vi "Export To File.vi"(4 "Always Overwrite":bool, 6 "Hide Grid":bool, 7 "Control Ref Queue":T1, 8 "error in (no error)":errorcluster, 9 "Path":path, 10 "Target":enum32{"File", "Clipboard"}(ring), 11 "File Type":enum32{"BMP", "EPS", "EMF", "PICT"}(ring)) -> (0 "error out":errorcluster)   [LabVIEW 2017, in "XY Plot Matrix.lvclass"]
uses:
  <vilib>/Math Plots/2D Math Plots/XY Plot Matrix/XY Plot Matrix/XY Plot Matrix.lvclass
  <vilib>/Math Plots/2D Math Plots/2D Plot/Action String/XYPlotMatrix Ctrl Act Queue.ctl
  <vilib>/Math Plots/2D Math Plots/2D Plot/Action String/XYPlotMatrix Ctrl Act Cluster.ctl
  <vilib>/Math Plots/2D Math Plots/2D Plot/Action String/2DMathPlot State Class.ctl
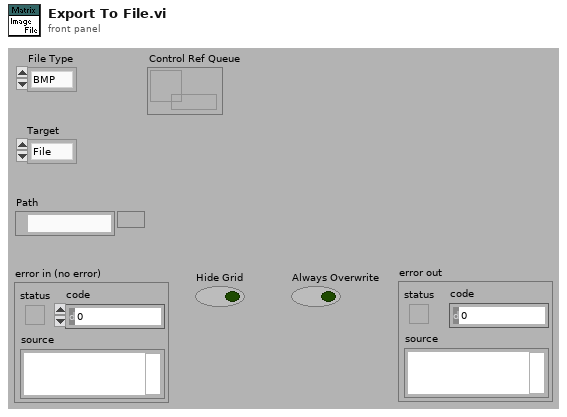
[diagram p1: front panel]
types:
  T1 = typedef "XYPlotMatrix Ctrl Act Queue.ctl" = refnum<queue>
  T2 = typedef "XYPlotMatrix Ctrl Act Cluster.ctl" = cluster{"Facade VI":refnum<vi>, "XControl":refnum<vi>, "Sub Panel":refnum<vi>, "Sub VI":refnum<vi>, "Export Image":refnum<vi>, "Display State Change Class":T3}
  T3 = typedef "2DMathPlot State Class.ctl" = enum16{"Update All (Undo)", "Update General", "Update Appearance", "Update Format", "Update Scale", "Update Marker", "Update Cursor", "None"}
  T4 = typedef "LVBoundsTypeDef.ctl" = cluster{"Width":u32, "Height":u32}
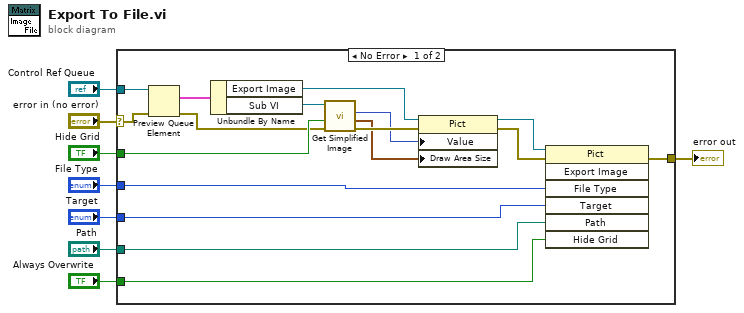
[diagram p0: block diagram]
diagram:
  n1 = case shown="No Error" "error in (no error)" {
    selector: "error in (no error)" -> [w11 w26]
    tunnel: "Hide Grid" -> [w21 _]
    tunnel: "Target" -> [w18 _]
    tunnel: "Path" -> [w17 _]
    tunnel: "File Type" -> [w9 _]
    tunnel: "Control Ref Queue" -> [w16 _]
    tunnel: [w13 w26] -> w3
    tunnel: "Always Overwrite" -> [w10 _]
    frame No Error {
      n2 = Preview Queue Element(queue=w16, error in (no error)=w11) -> (element=w15:T2, error out=w20:errorcluster)  [unwired: 3 out]
      n3 = Unbundle By Name(w15) -> ("Export Image"=w12:refnum<vi>, "Sub VI"=w19:refnum<vi>)
      n4 = call <vilib>:"Get Simplified Image.vi"("error in (no error)"=w20, "Hide Grid?"=w21, "Sub VI Ref"=w19) -> ("error out"=w24:errorcluster, "bounds"=w23:T4, "new picture"=w22:picture)  [unwired: 2 in, 4 out]
      n5 = property on="Property Node" class="Pict"(reference=w12, error in=w24, "Value"=w22, "Draw Area Size"=w23) -> (reference out=w14:refnum<vi>, error out=w25:errorcluster)
      n6 = invoke on="Invoke Node" class="Pict" method="Export Image"(reference=w14, error in=w25, "File Type"=w9, "Target"=w18, "Path"=w17, "Hide Grid"=w10) -> (error out=w13:errorcluster)  [unwired: 1 in, 6 out]
    }
    frame Error {
    }
  }
  "error out" <- w3
